vi "p2.vi"() -> ()   [LabVIEW 2021, in "d11.lvlib"]
uses:
  d11.lvlib
  5e485d29-ee1b-4304-9e56-c790280ef3da.vi
  <vilib>/Comparison/Less/Less Functor/Less Functor.lvclass
  AOC/AOC.lvlib
  <vilib>/gmath/NI_Gmath.lvlib
panel:
  out "Monkeys":T1(array[cluster])
  in  "Example":string="Monkey 0:\n  Starting items: 79, 98\n  Operation: new = old * 19\n  Test: divisible by 23\n    If true: throw to monkey 2\n    If false: throw to monkey 3\n\nMonkey 1:\n  Starting items: 54, 65, 75, 74\n  Operation: new = old + 6\n  Test: divisible by 19\n    If true: throw to monkey 2\n    If false: throw to monkey 0\n\nMonkey 2:\n  Starting items: 79, 60, 97\n  Operation: new = old * old\n  Test: divisible by 13\n    If true: throw to monkey 1\n    If false: throw to monkey 3\n\nMonkey 3:\n  Starting items: 74\n  Operation: new = old + 3\n  Test: divisible by 17\n    If true: throw to monkey 0\n    If false: throw to monkey 1"
  in  "Example":bool
  out "Answer":i64
  # "e"
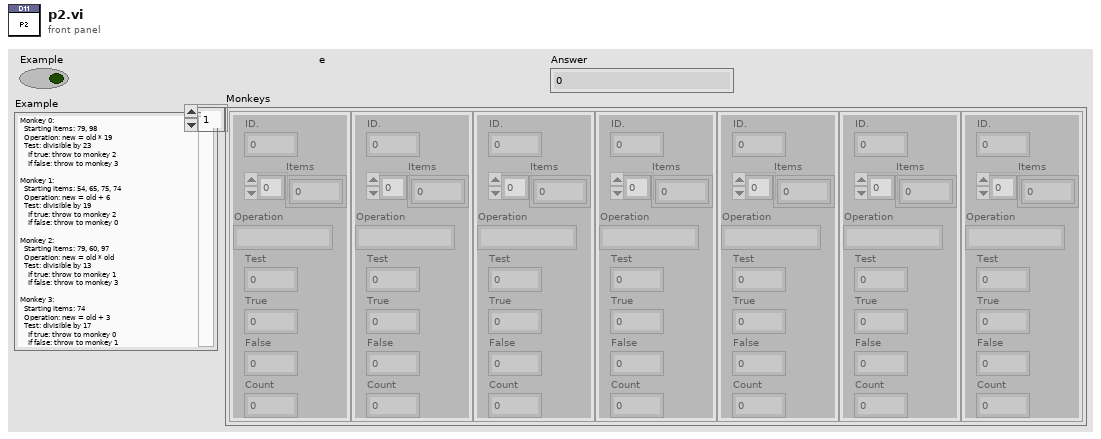
[diagram p1: front panel]
types:
  T1 = cluster{"ID.":i64, "Items":i64[], "Operation":string, "Test":i64, "True":i64, "False":i64, "Count":i64}[]
  T2 = cluster{"ID.":u64, "Items":i64[], "Operation":string, "Test":u64, "True":u64, "False":u64, "Count":u64}
  T3 = cluster{"ID.":u64, "Items":i64[], "Operation":string, "Test":u64, "True":u64, "False":u64, "Count":u64}[]
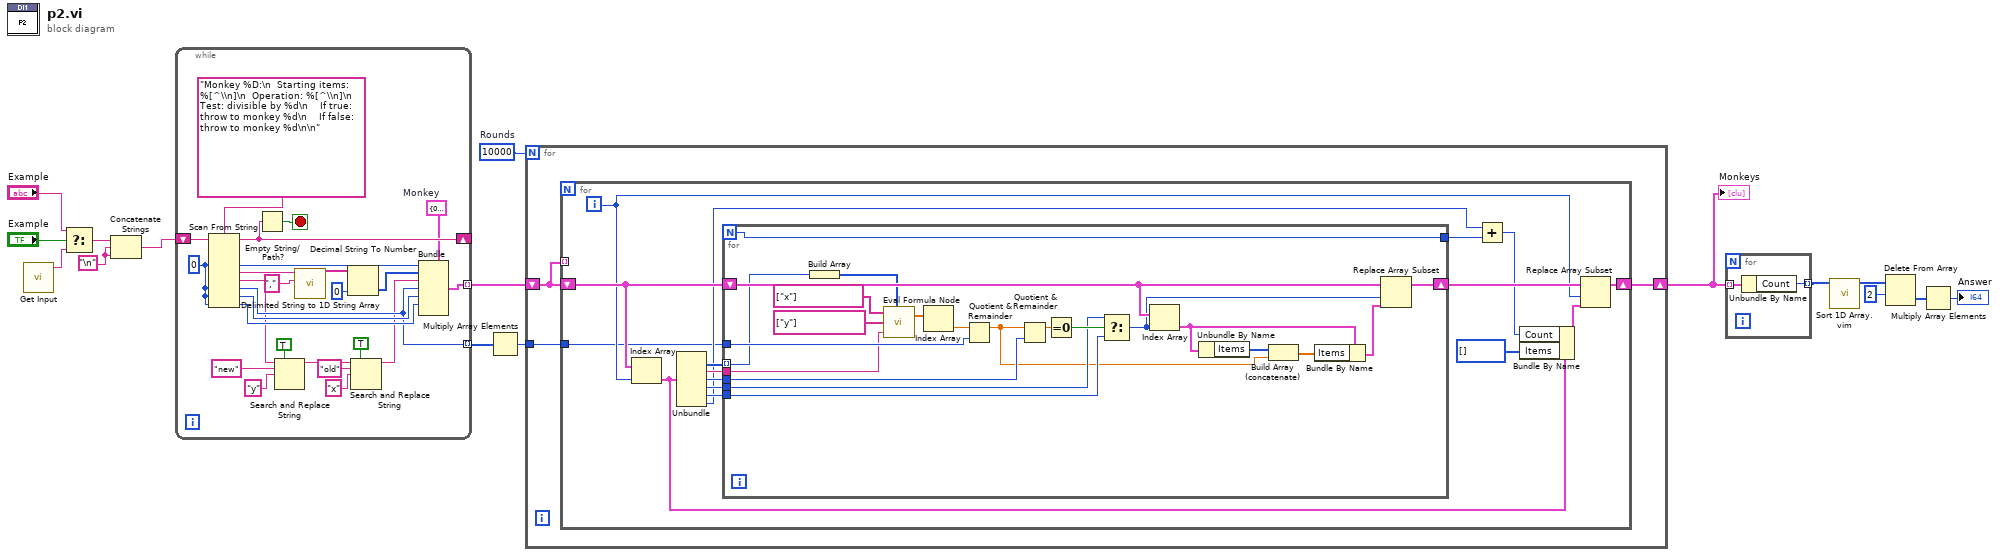
[diagram p0: block diagram]
diagram:
  w9 = "\n"
  w11 = 10000  # Rounds
  n1 = call "Get Input.vi"() -> ("Input"=w16:string)  [unwired: 11 in]
  n2 = Select(t="Example", s="Example", f=w16) -> (s? t:f=w13:string)
  n3 = Concatenate Strings(w13, w9, w9) -> (w10:string)
  n4 = while {
    shift-right: [w39] -> _
    shift-left: w10 -> [w41]
    tunnel: [w32] -> w12 mode=indexing
    tunnel: [w27] -> w2 mode=indexing
    stop <- w40 stop-if-true
    w29 = u64 0 ("default value 1")
    w30 = T2 {"ID."=0, "Items"=[], "Operation"="", "Test"=0, "True"=0, "False"=0, "Count"=0}  # Monkey
    n5 = Scan From String(format string="Monkey %D:\n  Starting items: %[^\\n]\n  Operation: %[^\\n]\n  Test: divisible by %d\n    If true: throw to monkey %d\n    If false: throw to monkey %d\n\n", input string=w41, default 1=w29, default 4=w29, default 5=w29, default 6=w29) -> (remaining string=w39:string, output 1=w36:u64, output 2=w37:string, output 3=w19:string, output 4=w27:u64, output 5=w34:u64, output 6=w33:u64)  [unwired: 4 in, 2 out]
    n6 = Empty String/Path?(string/path=w39) -> (empty?=w40:bool)
    n7 = Search and Replace String(replace all?=TRUE ("replace all? (F)"), input string=w19, search string="new" ("input string"), replace string="y" ("replace string (\"\")")) -> (result string=w24:string)  [unwired: 4 in, 3 out]
    n8 = call <vilib>:"Delimited String to 1D String Array.vi"("delimiter"=",", "delimited string"=w37) -> ("string array"=w35:string[])  [unwired: 9 in]
    n9 = Decimal String To Number(string=w35, default (0L)=i64 0 ("default (0 I32)")) -> (number=w31:i64[])  [unwired: 1 in, 1 out]
    n10 = Search and Replace String(replace all?=TRUE ("replace all? (F)"), input string=w24, search string="old", replace string="x" ("replace string (\"\")")) -> (result string=w18:string)  [unwired: 4 in, 3 out]
    n11 = Bundle(cluster=w30, "ID."=w36, "Items"=w31, "Operation"=w18, "Test"=w27, "True"=w34, "False"=w33) -> (w32:T2)  [unwired: 1 in]
  }
  n12 = Multiply Array Elements(1:w2) -> (0:w1:u64)
  n13 = for {
    N: w11 -> [_]
    shift-right: [w43] -> w8
    shift-left: w12 -> [w44]
    tunnel: w1 -> [w42]
    n14 = for {
      shift-right: [w52] -> w43
      shift-left: w44 -> [w55]
      tunnel: w44 -> [_] mode=indexing
      tunnel: w42 -> [w45]
      i -> [w50]
      n15 = Index Array(array=w55, index=w50) -> (element=w49:T2)
      n16 = Unbundle(w49) -> ("Items"=w59:i64[], "Operation"=w60:string, "Test"=w58:u64, "True"=w57:u64, "False"=w56:u64, "Count"=w47:u64)  [unwired: 1 out]
      n17 = for {
        N -> [w71]
        tunnel: w60 -> [w61]
        tunnel: w59 -> [w62] mode=indexing
        tunnel: w58 -> [w70]
        tunnel: w57 -> [w80]
        tunnel: w56 -> [w79]
        shift-right: [w76] -> w53
        shift-left: w55 -> [w77]
        tunnel: [w71] -> w48
        tunnel: w45 -> [w69]
        n18 = Build Array(w62) -> (w65:i64[])
        n19 = call <vilib>:"Eval Formula Node.vi"("Variables Input"=string[] ["x"], "Input Values"=w65, "Variables Output"=string[] ["y"], "formula"=w61) -> ("Output Values"=w64:dbl[])  [unwired: 1 in, 1 out]
        n20 = Index Array(array=w64) -> (element=w63:dbl)  [unwired: 1 in]
        n21 = Quotient & Remainder(x=w63, y=w69) -> (x-y*floor(x/y)=w68:dbl)  [unwired: 1 out]
        n22 = Quotient & Remainder(x=w68, y=w70) -> (x-y*floor(x/y)=w82:dbl)  [unwired: 1 out]
        n23 = Equal To 0?(x=w82) -> (x = 0?=w81:bool)
        n24 = Select(t=w80, s=w81, f=w79) -> (s? t:f=w75:u64)
        n25 = Index Array(array=w77, index=w75) -> (element=w74:T2)
        n26 = Unbundle By Name(w74) -> ("Items"=w78:i64[])
        n27 = Build Array (concatenate)(w78, w68) -> (w73:dbl[])
        n28 = Bundle By Name(cluster=w74, "Items"=w73) -> (w72:T2)
        n29 = Replace Array Subset(array=w77, new element=w72, index=w75) -> (w76:T3)
      }
      n30 = Add(x=w47, y=w48) -> (x+y=w46:u64)
      n31 = Bundle By Name(cluster=w49, "Count"=w46, "Items"=i64[] []) -> (w51:T2)
      n32 = Replace Array Subset(array=w53, new element=w51, index=w50) -> (w52:T3)
    }
  }
  "Monkeys" <- w8
  n33 = for {
    tunnel: w8 -> [w84] mode=indexing
    tunnel: [w83] -> w7 mode=indexing
    n34 = Unbundle By Name(w84) -> ("Count"=w83:u64)
  }
  n35 = call "Sort 1D Array.vim"("unsorted array"=w7) -> ("sorted array"=w6:u64[])  [unwired: 10 in]
  n36 = Delete From Array(array=w6, length=2) -> (deleted portion=w3:u64[])  [unwired: 1 in, 1 out]
  n37 = Multiply Array Elements(1:w3) -> (0:→"Answer":u64)
